vi "niRFSG Close.vi"(0 "instrument handle":refnum<k15>, 11 "error in":errorcluster {"code" format="%.0x"}) -> (15 "error out":errorcluster {"code" format="%.0x"})   [LabVIEW 2014]
doc: "Aborts any signal generation in progress and destroys the instrument driver session.\n\n<B>Supported Devices</B>: NI 5610/5611, NI 5644R/5645R/5646R, NI 5650/5651/5652/5654/5654 with NI 5696, NI 5670/5671/5672/5673/5673E, NI 5840"
uses:
  niRFSG.dll
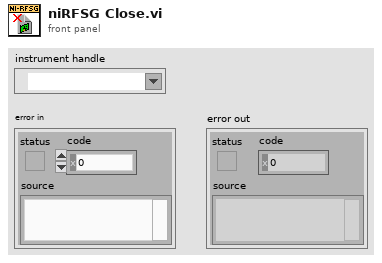
[diagram p1: front panel]
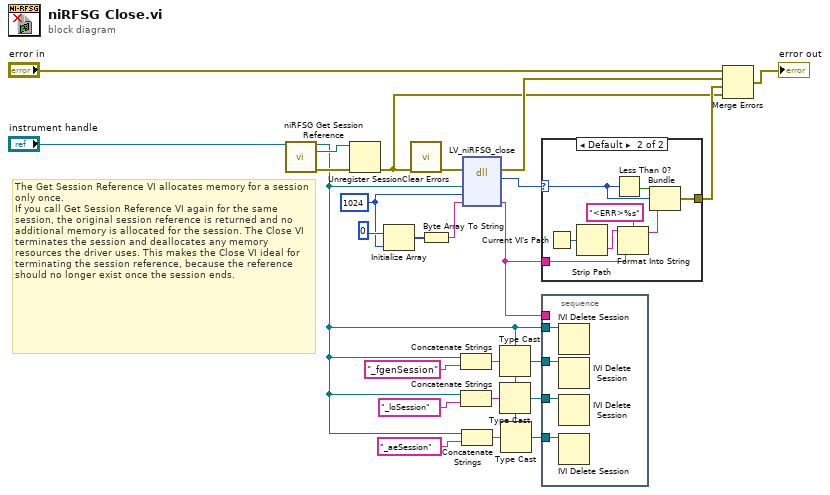
[diagram p0: block diagram]
diagram:
  w22 = 1024
  # "The Get Session Reference VI allocates memory for a session only once.\nIf you call Get Session Reference VI again for the same session, the original session reference is returned and no additional memory is allocated for the session. The Close VI terminates the session and deallocates any memory resources the driver uses. This makes the Close VI ideal for terminating the session reference, because the reference should no longer exist once the session ends."
  n1 = call "niRFSG Get Session Reference.vi"("instrument handle"="instrument handle") -> ("instrument handle out"=w5:refnum<k15>, "session reference"=w7:refnum<k20>, "error out"=w6:errorcluster)  [unwired: 12 in]
  n2 = Unregister Session(8:w6, 11:w7) -> (0:w2:errorcluster)
  n3 = Initialize Array(u8 0, w22) -> (w24:u8[])
  n4 = call "Clear Errors.vi"("error in (no error)"=w2) -> ("error out"=w4:errorcluster)  [unwired: 5 in, 1 out]
  n5 = Byte Array To String(unsigned byte array=w24) -> (string=w23:string)
  n6 = Concatenate Strings(w5, "_fgenSession" ("resource name (\"\")")) -> (w20:string)
  n7 = Concatenate Strings(w5, "_loSession" ("string")) -> (w17:string)
  n8 = Concatenate Strings(w5, "_aeSession" ("string")) -> (w11:string)
  n9 = dll-call lib="niRFSG**.*" fn="LV_niRFSG_close"(error in=w4, "instrument handle"=w5, "buffer size"=w22, "error buffer"=w23) -> (error out=w13:errorcluster, "status"=w3:i32, "error buffer"=w18:string)  [unwired: 4 in, 1 out]
  n10 = Type Cast(type=w5, x=w20) -> (*(type *) &x=w19:refnum<k15>)
  n11 = Type Cast(type=w5, x=w17) -> (*(type *) &x=w10:refnum<k15>)
  n12 = Type Cast(type=w5, x=w11) -> (*(type *) &x=w9:refnum<k15>)
  n13 = case shown="Default" w3 {
    selector: w3 -> [_ w26]
    tunnel: w18 -> [_ w31]
    tunnel: [_ w27] -> w14
    frame 0 {
    }
    frame Default {
      n14 = Current VI's Path() -> (path=w33:path)
      n15 = Strip Path(path=w33) -> (name=w32:string)  [unwired: 1 out]
      n16 = Less Than 0?(x=w26) -> (x < 0?=w28:bool)
      n17 = Format Into String(format string="<ERR>%s" ("Format String"), initial string=w32, w31) -> (resulting string=w29:string)  [unwired: 1 in, 1 out]
      n18 = Bundle(w28, "status"=w26, w29) -> (w27:cluster{bool, "status":i32, string})  [unwired: 1 in]
    }
  }
  n19 = stacked-sequence {
    tunnel: w5 -> [w37]
    tunnel: w19 -> [w36]
    tunnel: w18 -> [_]
    tunnel: w10 -> [w35]
    tunnel: w9 -> [w34]
    frame #0 {
      n20 = IVI Delete Session(11:w37) -> ()
      n21 = IVI Delete Session(11:w36) -> ()
      n22 = IVI Delete Session(11:w35) -> ()
      n23 = IVI Delete Session(11:w34) -> ()
    }
  }
  n24 = Merge Errors("error in", w13, w14, w2) -> (→"error out":errorcluster)
